vi "Dashboard Main 2.vi"() -> ()   [LabVIEW 2012]
uses:
  <vilib>/Rock Robotics/WPI/Camera/WPI_CameraImageSize.ctl
  <vilib>/Utility/config.llb/Read Key (String).vi
  <vilib>/Utility/config.llb/Read Key (I32).vi
  <vilib>/Utility/config.llb/Write Key (String).vi
  <vilib>/Utility/config.llb/Write Key (I32).vi
  <vilib>/Rock Robotics/WPI/Camera/WPI_CameraSettings Read MJPG.ctl
  <vilib>/Utility/config.llb/NI_LVConfig.lvlib
panel:
  in  "Camera Settings 2":T1={"Frate Rate"=30, "Compression"=30, "Size"=1} {"Frate Rate" scale=1.0..30.0; "Size" items=["640x480", "320x240", "160x120"]}
  in  "DB Camera Config":bool
  in  "Enable":bool
  out "Camera Image":T2(plugin-control)
  out "Mbps":dbl format="%#.1g"
  out "fps":dbl format="%#.1g"
  out "Camera Image 2":T2(plugin-control)
  in  "Camera Settings":T1={"Frate Rate"=30, "Compression"=30, "Size"=1} {"Frate Rate" scale=1.0..30.0; "Size" items=["640x480", "320x240", "160x120"]}
  in  "Enable Camera":bool
  in  "Image Size":T3
  in  "Compression":dbl(slide) min=0.0 max=100.0 scale=0.0..100.0
  in  "FPS":dbl(slide) scale=10.0..30.0
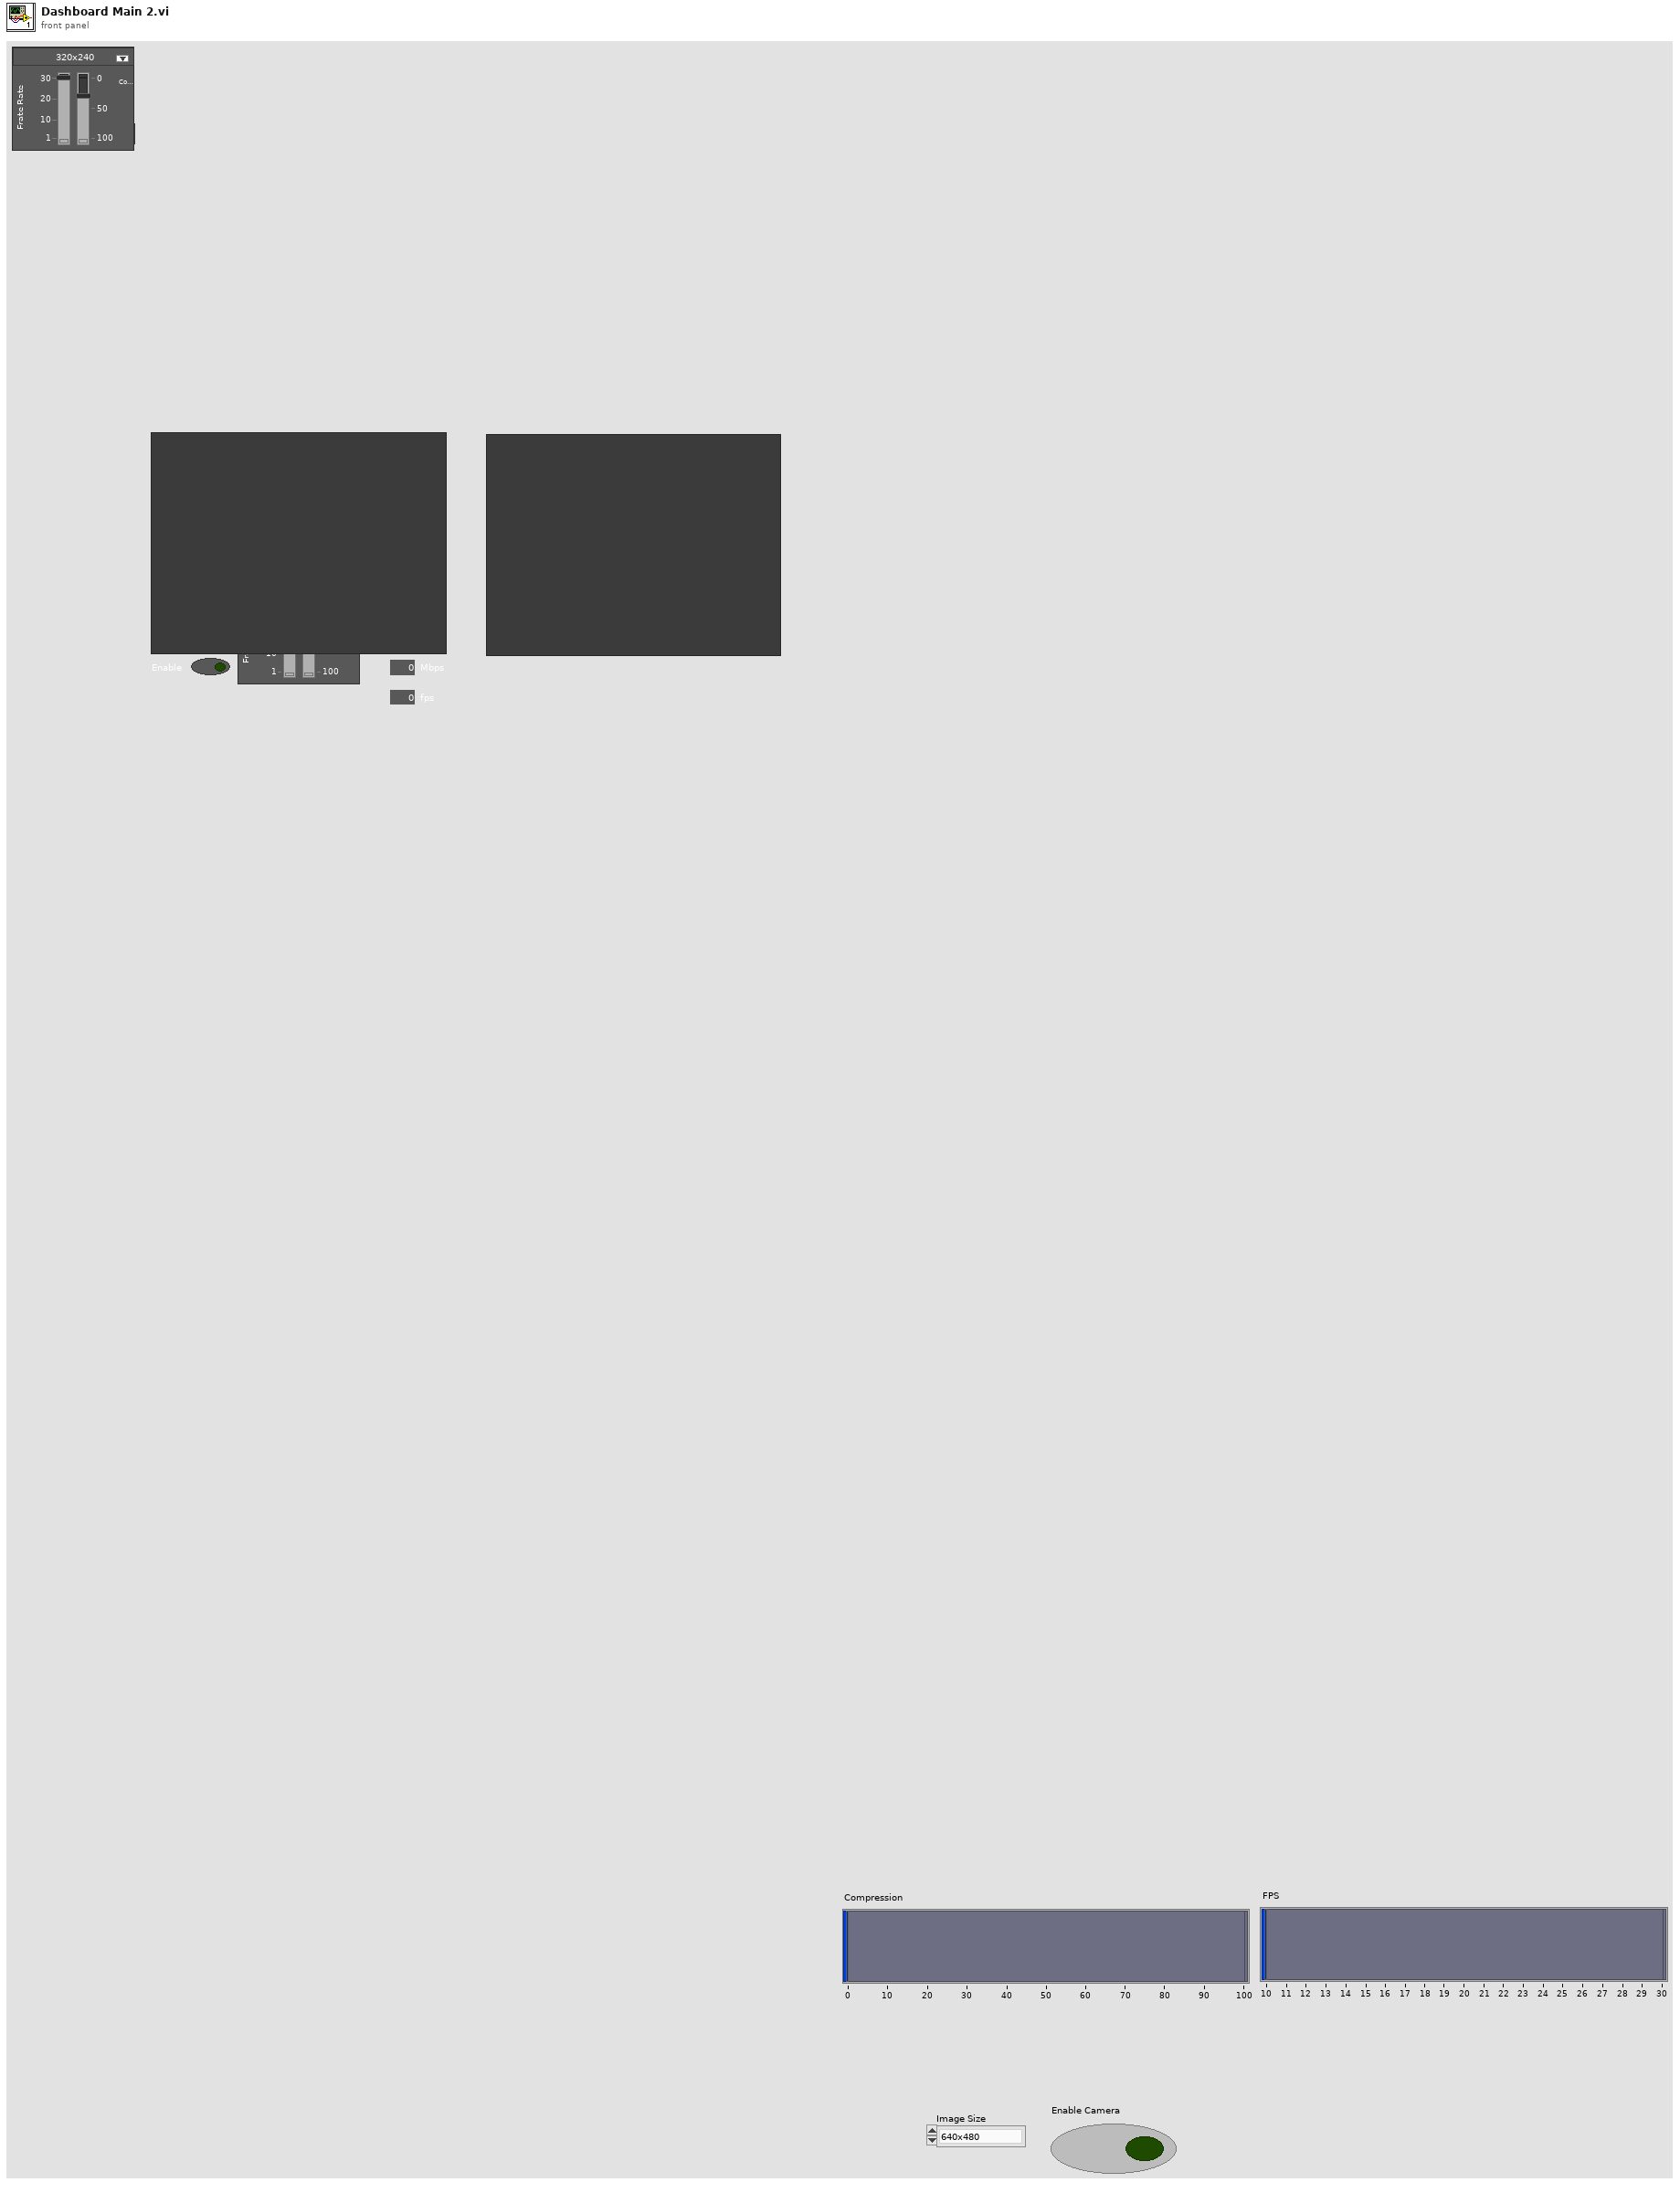
[diagram p1: front panel]
types:
  T1 = cluster{"Frate Rate":i32, "Compression":i32, "Size":u16}
  T2 = typedef "IMAQ Image.ctl" = refnum<image>
  T3 = typedef "WPI_CameraImageSize.ctl" = enum16{"640x480", "320x240", "160x120"}
  T4 = typedef "Image Type" = u32
  T5 = typedef "NI_LVConfig.lvlib/Config Data RefNum.ctl" = refnum<k1>
  T6 = typedef "LVRectTypeDef.ctl" = cluster{"Left":i16, "Top":i16, "Right":i16, "Bottom":i16}
  T7 = typedef "WPI_CameraSettings Read MJPG.ctl" = cluster{"fps":i32, "compression":i32, "Image Size":T3}
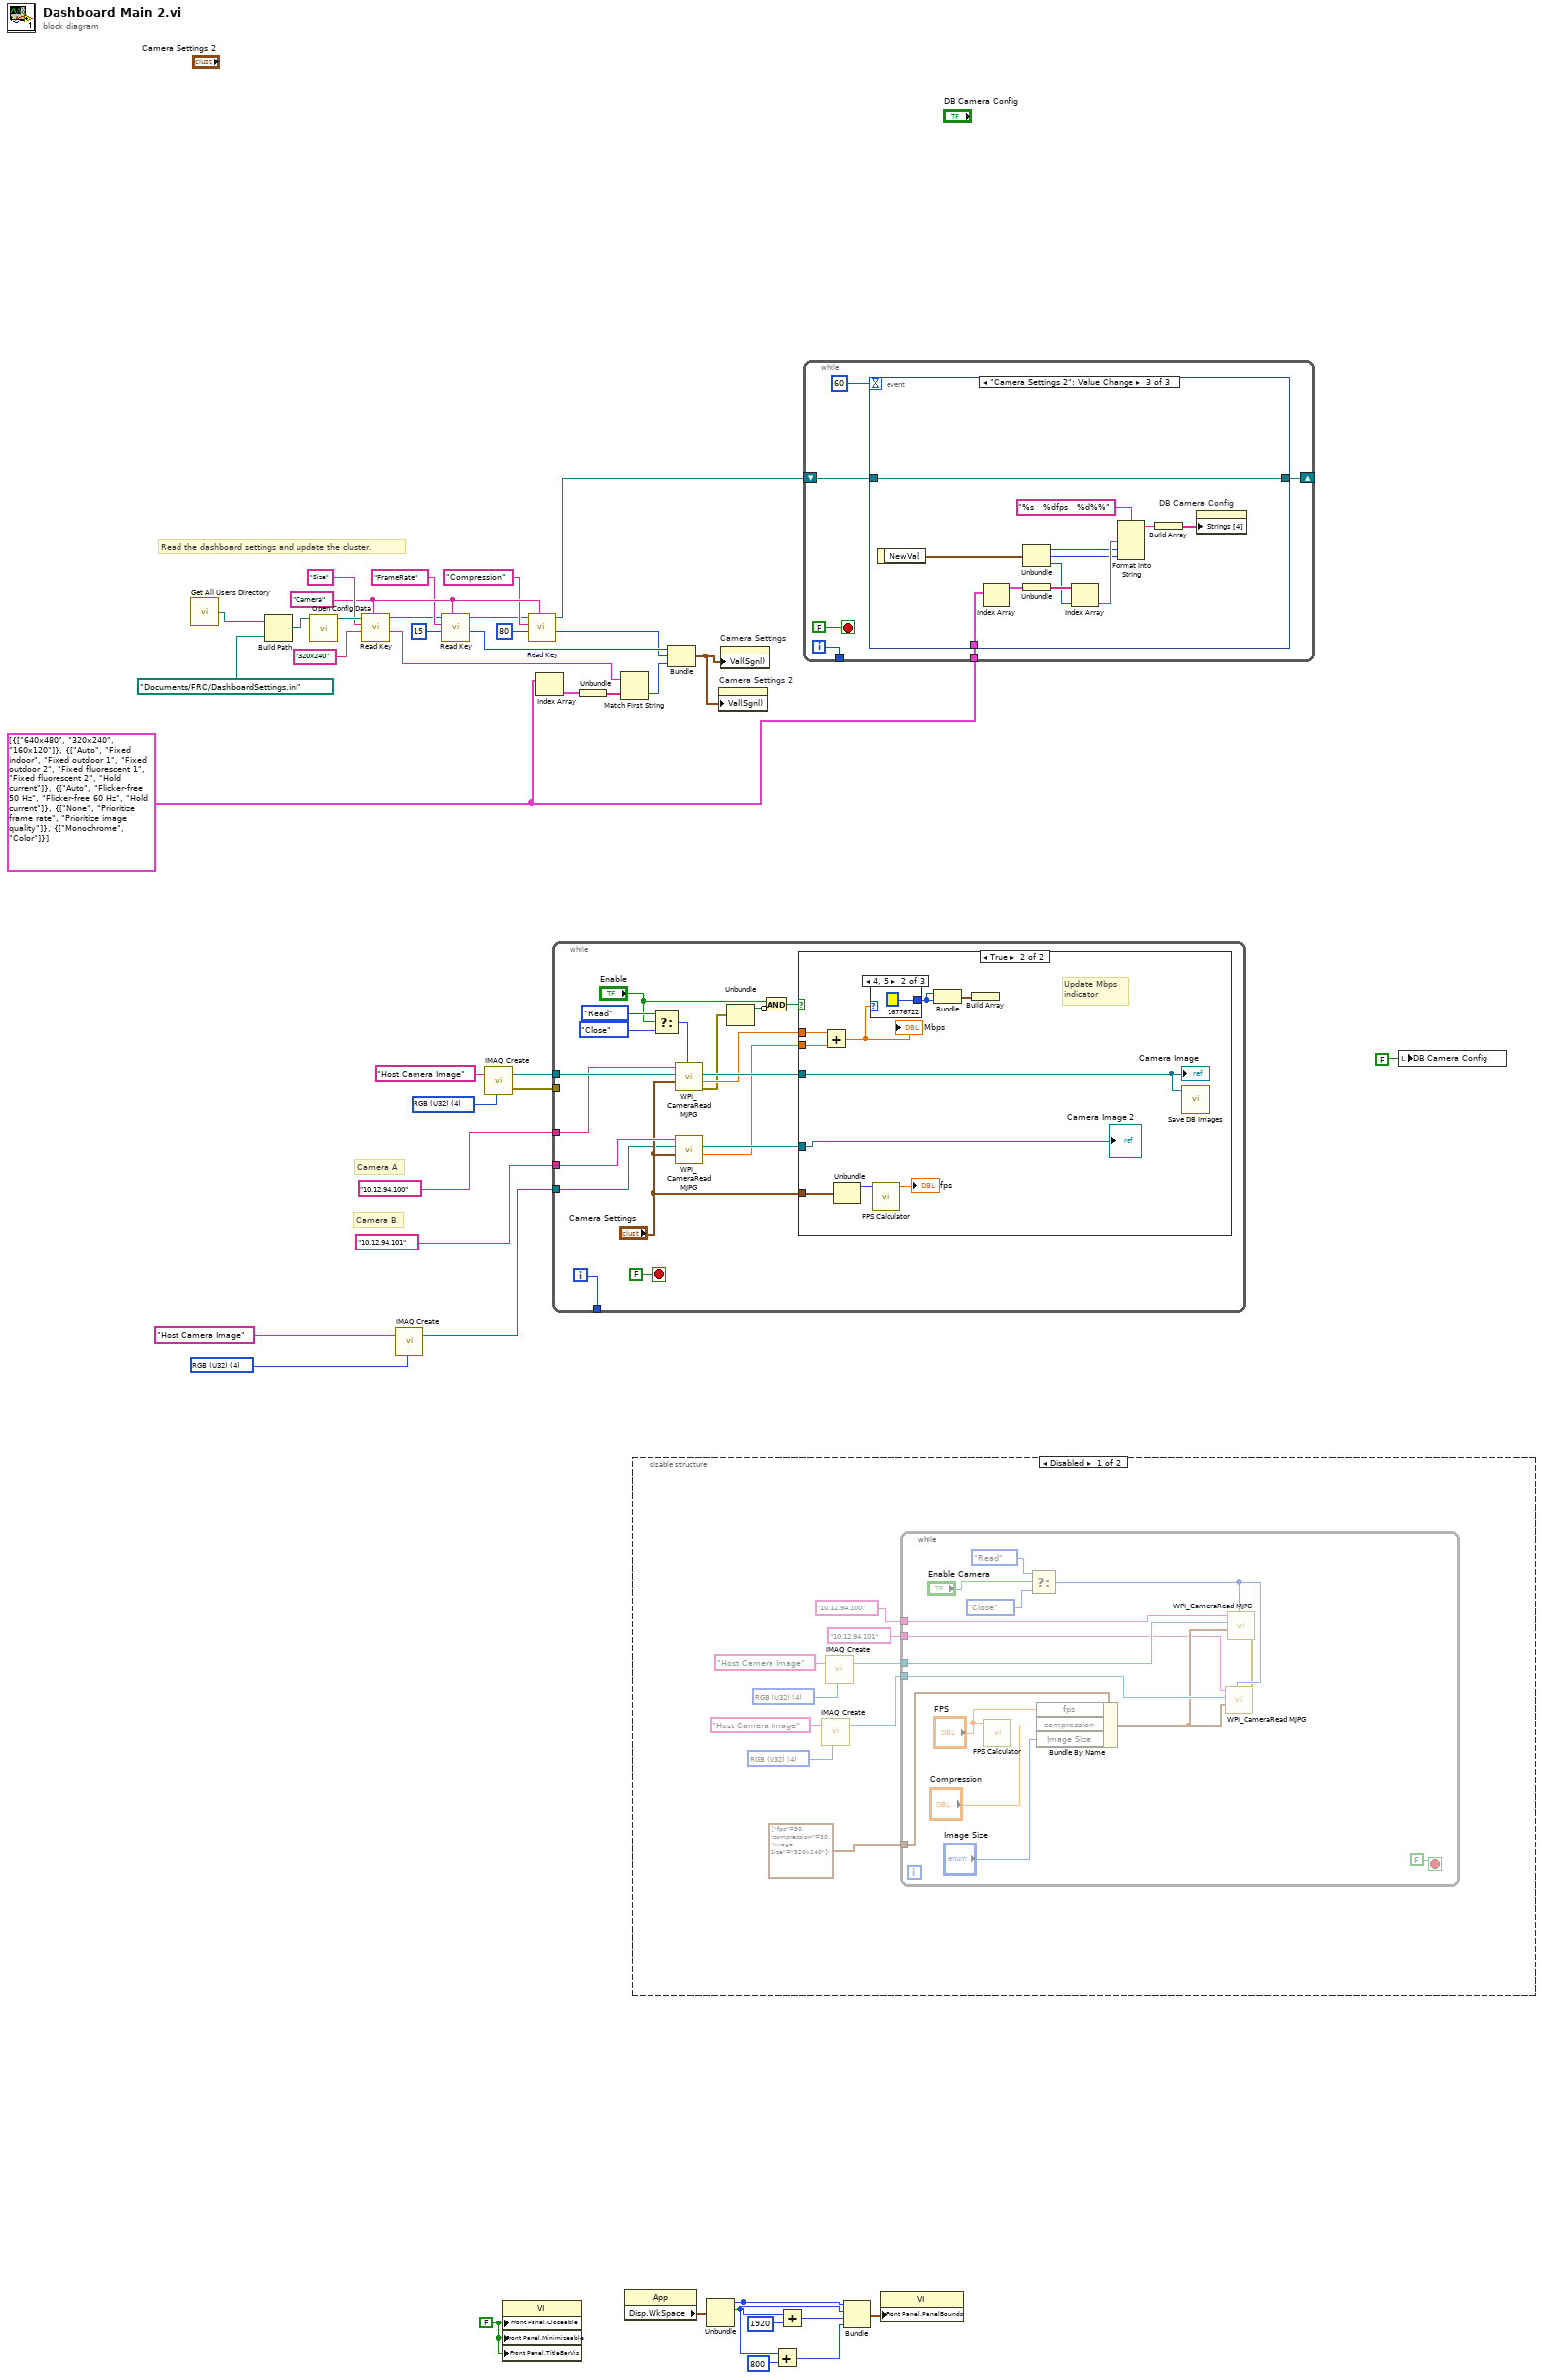
[diagram p0: block diagram]
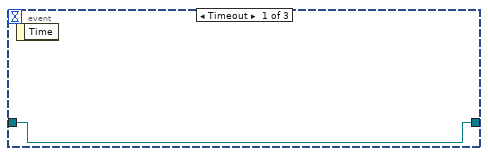
[diagram p2: hidden frame]
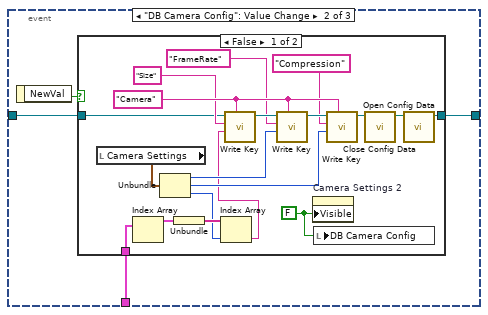
[diagram p3: hidden frame]
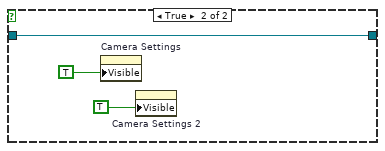
[diagram p4: hidden frame]
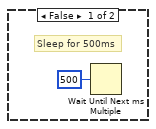
[diagram p6: hidden frame]
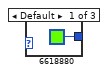
[diagram p7: hidden frame]
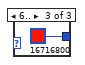
[diagram p8: hidden frame]
diagram:
  w17 = "Camera"
  w2 = cluster{string[]}[] [{["640x480", "320x240", "160x120"]}, {["Auto", "Fixed indoor", "Fixed outdoor 1", "Fixed outdoor 2", "Fixed fluorescent 1", "Fixed fluorescent 2", "Hold current"]}, {["Auto", "Flicker-free 50 Hz", "Flicker-free 60 Hz", "Hold current"]}, {["None", "Prioritize frame rate", "Prioritize image quality"]}, {["Monochrome", "Color"]}]
  w26 = T4 4 items=["Grayscale (U8)", "Grayscale (I16)", "Grayscale (SGL)", "Complex (CSG)", "RGB (U32)", "HSL (U32)", "RGB (U64)"] ("Image Type")
  w32 = T4 4 items=["Grayscale (U8)", "Grayscale (I16)", "Grayscale (SGL)", "Complex (CSG)", "RGB (U32)", "HSL (U32)", "RGB (U64)"] ("Image Type")
  w41 = FALSE ("Front Panel Window:Closeable")
  # "Read the dashboard settings and update the cluster."
  # "Camera B"
  # "Camera A"
  n1 = call "Get All Users Directory.vi"() -> ("All User Path"=w22:path)
  n2 = Build Path(base path=w22, name or relative path=path "Documents/FRC/DashboardSettings.ini") -> (appended path=w21:path)
  n3 = call <vilib>:"Open Config Data.vi"("configuration file path"=w21) -> ("refnum"=w20:T5)  [unwired: 8 in, 2 out]
  n4 = call-poly <vilib>:"Read Key.vi"("section"=w17, "default value"="320x240", "key"="Size", "refnum"=w20) -> ("value"=w8:string, "refnum out"=w5:T5)  [unwired: 2 in, 4 out]
  n5 = call "IMAQ Create"("Image Name"="Host Camera Image", "Image Type"=w26) -> ("New Image"=w24:T2)  [unwired: 2 in, 2 out]
  n6 = call-poly <vilib>:"Read Key.vi"("section"=w17, "default value"=15, "key"="FrameRate", "refnum"=w5) -> ("value"=w12:i32, "refnum out"=w4:T5)  [unwired: 1 in, 5 out]
  n7 = call "IMAQ Create"("Image Name"="Host Camera Image", "Image Type"=w32) -> ("New Image"=w30:T2, "error out"=w29:errorcluster)  [unwired: 2 in, 1 out]
  n8 = property class="VI"("Front Panel.Closeable"=w41, "Front Panel.Minimizeable"=w41, "Front Panel.TitleBarVis"=w41) -> ()  [unwired: 2 in, 2 out]
  n9 = call-poly <vilib>:"Read Key.vi"("section"=w17, "default value"=80, "key"="Compression", "refnum"=w4) -> ("value"=w11:i32, "refnum out"=w3:T5)  [unwired: 1 in, 5 out]
  n10 = Index Array(array=w2) -> (element=w10:cluster{string[]})  [unwired: 1 in]
  n11 = while {
    tunnel: w30 -> [w57]
    tunnel: w29 -> [_]
    tunnel: [w58] -> _
    tunnel: "10.12.94.100" -> [w43]
    tunnel: "10.12.94.101" -> [w45]
    tunnel: w24 -> [w42]
    i -> [w58]
    stop <- FALSE stop-if-true
    n12 = Select(t=enum16{"Read", "Reopen", "Close"}."Read" ("Operation"), s="Enable", f=enum16{"Read", "Reopen", "Close"}."Close" ("Operation")) -> (s? t:f=w52:enum16{"Read", "Reopen", "Close"})
    n13 = call <vilib>:"WPI_CameraRead MJPG.vi"("Operation"=w52, "Camera Settings"="Camera Settings", "Image"=w57, "address"=w43) -> ("error out"=w51:errorcluster, "Bandwidth (kbps)"=w55:dbl, "Image Out"=w56:T2)  [unwired: 5 in]
    n14 = call <vilib>:"WPI_CameraRead MJPG.vi"("Camera Settings"="Camera Settings", "Image"=w42, "address"=w45) -> ("Bandwidth (kbps)"=w46:dbl, "Image Out"=w47:T2)  [unwired: 6 in, 1 out]
    n15 = Unbundle(w51) -> ("status"=w49:bool)  [unwired: 2 out]
    n16 = Compound Arithmetic op=AND("Enable", invert w49) -> (w48:bool)
    n17 = case shown="True" w48 {
      tunnel: "Camera Settings" -> [_ w67]
      tunnel: w56 -> [_ w65]
      tunnel: w55 -> [_ w63]
      tunnel: w47 -> [_ w61]
      tunnel: w46 -> [_ w64]
      frame False {
        # "Sleep for 500ms"
        n18 = Wait Until Next ms Multiple(millisecond multiple=u32 500) -> ()  [unwired: 1 out]
      }
      frame True {
        # "Update Mbps\nindicator"
        n19 = Add(x=w63, y=w64) -> (x+y=w62:dbl)
        "Mbps" <- w62
        n20 = Unbundle(w67) -> ("Frate Rate"=w66:i32)  [unwired: 2 out]
        n21 = case shown="4, 5" w62 {
          tunnel: [u32 6618880 ("Color Box") u32 16776722 ("Color Box") u32 16716800 ("Color Box")] -> w69
          frame Default {
          }
          frame 4, 5 {
          }
          frame 6.. {
          }
        }
        n22 = call "FPS Calculator.vi"("Average Count"=w66) -> ("fps"=→"fps":dbl)  [unwired: 10 in]
        n23 = Bundle("Color Box"=w69, "Color Box"=w69) -> (w70:cluster{"Color Box":u32, "Color Box":u32})  [unwired: 1 out]
        n24 = Build Array(w70) -> ()  [unwired: 1 out]
        n25 = call "Save DB Images.vi"("Image"=w65) -> ()  [unwired: 2 in, 1 out]
        "Camera Image" <- w65
        "Camera Image 2" <- w61
      }
    }
  }
  n26 = Unbundle(w10) -> (w9:string[])
  n27 = Match First String(2:w9, 3:w8) -> (0:w7:i32)  [unwired: 1 out]
  n28 = property class="App"() -> ("Disp.WkSpace"=w39:T6)  [unwired: 2 in, 2 out]
  n29 = disable-structure shown="Disabled" {
    frame Disabled {
      w76 = T4 4 items=["Grayscale (U8)", "Grayscale (I16)", "Grayscale (SGL)", "Complex (CSG)", "RGB (U32)", "HSL (U32)", "RGB (U64)"] ("Image Type")
      w81 = T4 4 items=["Grayscale (U8)", "Grayscale (I16)", "Grayscale (SGL)", "Complex (CSG)", "RGB (U32)", "HSL (U32)", "RGB (U64)"] ("Image Type")
      n30 = call "IMAQ Create"("Image Name"="Host Camera Image", "Image Type"=w76) -> ("New Image"=w74:T2)  [unwired: 2 in, 2 out]
      n31 = call "IMAQ Create"("Image Name"="Host Camera Image", "Image Type"=w81) -> ("New Image"=w79:T2)  [unwired: 2 in, 2 out]
      n32 = while {
        tunnel: "10.12.94.101" ("address") -> [w83]
        tunnel: w79 -> [w98]
        tunnel: T7 {"fps"=30, "compression"=30, "Image Size"=enum."320x240"} ("Camera Settings") -> [w97]
        tunnel: "10.12.94.100" ("address") -> [w84]
        tunnel: w74 -> [w86]
        stop <- FALSE stop-if-true
        n33 = call "FPS Calculator.vi"("Average Count"="FPS") -> ()  [unwired: 10 in, 1 out]
        n34 = Select(t=enum16{"Read", "Reopen", "Close"}."Read" ("Operation"), s="Enable Camera", f=enum16{"Read", "Reopen", "Close"}."Close" ("Operation")) -> (s? t:f=w90:enum16{"Read", "Reopen", "Close"})
        n35 = Bundle By Name(cluster=w97, "fps"="FPS", "compression"="Compression", "Image Size"="Image Size") -> (w85:T7)
        n36 = call <vilib>:"WPI_CameraRead MJPG.vi"("Operation"=w90, "Camera Settings"=w85, "Image"=w98, "address"=w84) -> ("error out"=w89:errorcluster, "Image Out"=w88:T2)  [unwired: 5 in, 1 out]
        n37 = call <vilib>:"WPI_CameraRead MJPG.vi"("Operation"=w90, "error in"=w89, "Camera Settings"=w85, "Image"=w86, "address"=w83) -> ("Image Out"=w87:T2)  [unwired: 4 in, 2 out]
      }
    }
    frame Enabled {
    }
  }
  n38 = Bundle("value"=w12, "value"=w11, "index"=w7) -> (w1:cluster{"value":i32, "value":i32, "index":i32})  [unwired: 1 out]
  n39 = Unbundle(w39) -> ("Left"=w33:i16, "Top"=w34:i16)  [unwired: 2 out]
  n40 = property on="Camera Settings 2" class="Clust (strict)"("Val(Sgnl)"=w1) -> ()  [unwired: 2 in, 2 out]
  n41 = property on="Camera Settings" class="Clust (strict)"("Val(Sgnl)"=w1) -> ()  [unwired: 2 in, 2 out]
  n42 = Add(x=w34, y=i16 800) -> (x+y=w37:i16)
  n43 = Add(x=w33, y=i16 1920) -> (x+y=w38:i16)
  n44 = while {
    tunnel: w2 -> [w103]
    shift-right: [w102] -> _
    shift-left: w3 -> [w101]
    tunnel: [w100] -> _
    i -> [w100]
    stop <- FALSE stop-if-true
    n45 = event shown="[2] \"Camera Settings 2\": Value Change" {
      selector: _ -> [_ _ _]
      dyn-events: _ -> [_ _ _]
      timeout: u32 60 ("milliseconds to wait") -> [_ _ _]
      tunnel: w103 -> [_ w109 w140]
      tunnel: [w106 w108 w133] -> w102
      tunnel: w101 -> [w106 w107 w133]
      event Timeout {
        n46 = event-data() -> ()  [unwired: 1 in, 1 out]
      }
      event "DB Camera Config": Value Change {
        n47 = event-data() -> ("NewVal"=w110:bool)  [unwired: 1 in]
        n48 = case shown="False" w110 {
          tunnel: w109 -> [w119 _]
          tunnel: [w112 w131] -> w108
          tunnel: w107 -> [w111 w131]
          frame False {
            w126 = "Camera"
            w129 = FALSE ("Visible")
            n49 = local read "Camera Settings"() -> (w118:T1)
            n50 = Index Array(array=w119) -> (element=w122:cluster{string[]})  [unwired: 1 in]
            n51 = Unbundle(w118) -> ("Frate Rate"=w117:i32, "Compression"=w116:i32, "Size"=w120:u16)
            n52 = Unbundle(w122) -> (w121:string[])
            n53 = Index Array(array=w121, index=w120) -> (element=w115:string)
            n54 = call-poly <vilib>:"Write Key.vi"("section"=w126, "value"=w115, "key"="Size", "refnum"=w111) -> ("refnum out"=w128:T5)  [unwired: 2 in, 5 out]
            n55 = call-poly <vilib>:"Write Key.vi"("section"=w126, "value"=w117, "key"="FrameRate", "refnum"=w128) -> ("refnum out"=w127:T5)  [unwired: 1 in, 6 out]
            n56 = property on="Camera Settings 2" class="Clust (strict)"("Visible"=w129) -> ()  [unwired: 2 in, 2 out]
            n57 = local write "DB Camera Config"(w129) -> ()
            n58 = call-poly <vilib>:"Write Key.vi"("section"=w126, "value"=w116, "key"="Compression", "refnum"=w127) -> ("refnum out"=w113:T5)  [unwired: 1 in, 6 out]
            n59 = call <vilib>:"Close Config Data.vi"("refnum"=w113) -> ("file path"=w114:path)  [unwired: 2 in, 8 out]
            n60 = call <vilib>:"Open Config Data.vi"("configuration file path"=w114) -> ("refnum"=w112:T5)  [unwired: 8 in, 2 out]
          }
          frame True {
            n61 = property on="Camera Settings" class="Clust (strict)"("Visible"=TRUE) -> ()  [unwired: 2 in, 2 out]
            n62 = property on="Camera Settings 2" class="Clust (strict)"("Visible"=TRUE) -> ()  [unwired: 2 in, 2 out]
          }
        }
      }
      event "Camera Settings 2": Value Change {
        n63 = event-data() -> ("NewVal"=w144:T1)  [unwired: 1 in]
        n64 = Index Array(array=w140) -> (element=w139:cluster{string[]})  [unwired: 1 in]
        n65 = Unbundle(w144) -> ("Frate Rate"=w135:i32, "Compression"=w134:i32, "Size"=w137:u16)
        n66 = Unbundle(w139) -> (w138:string[])
        n67 = Index Array(array=w138, index=w137) -> (element=w136:string)
        n68 = Format Into String(format string="%s   %dfps   %d%%", w136, w135, w134) -> (resulting string=w141:string)  [unwired: 2 in, 1 out]
        n69 = Build Array(w141) -> (w142:string[])
        n70 = property on="DB Camera Config" class="Bool (strict)"("Strings [4]"=w142) -> ()  [unwired: 2 in, 2 out]
      }
    }
  }
  n71 = Bundle("Left"=w33, "Top"=w34, w38, w37) -> (w40:cluster{"Left":i16, "Top":i16, i16, i16})  [unwired: 1 out]
  n72 = property class="VI"("Front Panel.PanelBounds"=w40) -> ()  [unwired: 2 in, 2 out]
  n73 = local write "DB Camera Config"(FALSE ("DB Camera Config")) -> ()
